vi "3d_aircraft.vi"(4 "RH Aileron":dbl=-2.3415980339050293 format="%#.4f", 5 "Elevator":dbl(slide)=4.274326801300049 scale=-10.0..10.0, 6 "LH Aileron":dbl=1.756198525428772 format="%#.4f", 7 "Rudder":dbl(slide)=-0.13481126725673676 scale=-10.0..10.0, 8 "Heading (deg)":dbl(knob) scale=0.0..360.0, 9 "Roll (deg)":dbl(slide)=61.490421295166016 scale=-40.0..40.0, 10 "Pitch (deg)":dbl(slide)=-8.517632484436035 scale=-20.0..20.0, 11 "visual":refnum<k7>(container) caption="3D 파라미터형 표면") -> ()   [LabVIEW 2015]
uses:
  <vilib>/express/express arith-compare/Formula/XNode/ExpressFormulaBlockNode.xnode
  <vilib>/Platform/NI_3dgraph.lvlib
panel:
  in  "Rudder z":dbl[][](array[numeric])=[[0.0, 0.0, 0.0, 0.0], [0.0, 0.4, 0.4, 0.0], [0.0, 1.1, 1.1, 0.0], [0.0, 1.5, 1.5, 0.0], [0.0, 1.4, 1.4, 0.0], [0.0, -1.4, -1.4, 0.0], [0.0, -1.5, -1.5, 0.0], [0.0, -1.1, -1.1, 0.0], [0.0, -0.4, -0.4, 0.0], [0.0, 0.0, 0.0, 0.0]]
  in  "Rudder y":dbl[][](array[numeric])=[[0.8, 7.0, 14.0, 21.0], [0.6, 7.0, 14.0, 21.0], [0.4, 7.0, 14.0, 21.0], [0.2, 7.0, 14.0, 21.0], [0.0, 7.0, 14.0, 21.0], [0.0, 7.0, 14.0, 21.0], [0.2, 7.0, 14.0, 21.0], [0.4, 7.0, 14.0, 21.0], [0.6, 7.0, 14.0, 21.0], [0.8, 7.0, 14.0, 21.0]]
  in  "Rudder x":dbl[][](array[numeric])=[[5.0, 5.0, 5.0, 5.0], [4.6667, 4.6667, 4.6667, 4.6667], [2.5, 2.5, 2.5, 2.5], [0.8333, 0.8333, 0.8333, 0.8333], [0.0, 0.0, 0.0, 0.0], [0.0, 0.0, 0.0, 0.0], [0.8333, 0.8333, 0.8333, 0.8333], [2.5, 2.5, 2.5, 2.5], [4.6667, 4.6667, 4.6667, 4.6667], [5.0, 5.0, 5.0, 5.0]]
  in  "Elevator z":dbl[][](array[numeric])=[[0.0, 0.0, 0.0, 0.0], [0.0, 0.4, 0.4, 0.0], [0.0, 1.1, 1.1, 0.0], [0.0, 1.5, 1.5, 0.0], [0.0, 1.4, 1.4, 0.0], [0.0, -1.4, -1.4, 0.0], [0.0, -1.5, -1.5, 0.0], [0.0, -1.1, -1.1, 0.0], [0.0, -0.4, -0.4, 0.0], [0.0, 0.0, 0.0, 0.0]]
  in  "Elevator y":dbl[][](array[numeric])=[[-12.0, -12.0, 12.0, 12.0], [-12.0, -12.0, 12.0, 12.0], [-12.0, -12.0, 12.0, 12.0], [-12.0, -12.0, 12.0, 12.0], [-12.0, -12.0, 12.0, 12.0], [-12.0, -12.0, 12.0, 12.0], [-12.0, -12.0, 12.0, 12.0], [-12.0, -12.0, 12.0, 12.0], [-12.0, -12.0, 12.0, 12.0], [-12.0, -12.0, 12.0, 12.0]]
  in  "Elevator x":dbl[][](array[numeric])=[[5.0, 5.0, 5.0, 5.0], [4.6667, 4.6667, 4.6667, 4.6667], [2.5, 2.5, 2.5, 2.5], [0.8333, 0.8333, 0.8333, 0.8333], [0.0, 0.0, 0.0, 0.0], [0.0, 0.0, 0.0, 0.0], [0.8333, 0.8333, 0.8333, 0.8333], [2.5, 2.5, 2.5, 2.5], [4.6667, 4.6667, 4.6667, 4.6667], [5.0, 5.0, 5.0, 5.0]]
  in  "Aileron z":dbl[][](array[numeric])=[[0.0, 0.0, 0.0, 0.0], [0.0, 0.3276, 0.3276, 0.0], [0.0, 0.5994, 0.5994, 0.0], [0.0, 1.0388, 1.0388, 0.0], [0.0, 1.3762, 1.3762, 0.0], [0.0, -0.2418, -0.2418, 0.0], [0.0, -0.1612, -0.1612, 0.0], [0.0, -0.0806, -0.0806, 0.0], [0.0, -0.0402, -0.0402, 0.0], [0.0, 0.0, 0.0, 0.0]]
  in  "Aileron y":dbl[][](array[numeric])=[[0.0, 0.0, 56.0, 56.0], [0.0, 0.0, 56.0, 56.0], [0.0, 0.0, 56.0, 56.0], [0.0, 0.0, 56.0, 56.0], [0.0, 0.0, 56.0, 56.0], [0.0, 0.0, 56.0, 56.0], [0.0, 0.0, 56.0, 56.0], [0.0, 0.0, 56.0, 56.0], [0.0, 0.0, 56.0, 56.0], [0.0, 0.0, 56.0, 56.0]]
  in  "Aileron x":dbl[][](array[numeric])=[[6.0, 6.0, 6.0, 6.0], [5.0, 5.0, 5.0, 5.0], [4.0, 4.0, 4.0, 4.0], [2.0, 2.0, 2.0, 2.0], [0.09999999999999964, 0.09999999999999964, 0.09999999999999964, 0.09999999999999964], [0.09999999999999964, 0.09999999999999964, 0.09999999999999964, 0.09999999999999964], [2.0, 2.0, 2.0, 2.0], [4.0, 4.0, 4.0, 4.0], [5.0, 5.0, 5.0, 5.0], [6.0, 6.0, 6.0, 6.0]]
  in  "Body z":dbl[][](array[numeric])=[[0.0, 0.0, 0.0, 0.0, 0.0, 0.0, 0.0, 0.0, 0.0], [-0.5, 1.0, 1.0, 20.0, 22.0, 20.0, 1.0, 1.0, -0.5], [-0.5, 1.5, 1.5, 20.0, 22.0, 20.0, 1.5, 1.5, -0.5], [-0.5, 1.0, 1.0, 8.0, 10.0, 8.0, 1.0, 1.0, -0.5], [-1.5, 0.0, 0.0, 3.0, 5.0, 3.0, 0.0, 0.0, -1.5], [-2.0, 0.0, 0.0, 0.0, 0.0, 0.0, 0.0, 0.0, -2.0], [-3.0, -0.276, -0.276, -0.276, -0.276, -0.276, -0.276, -0.276, -2.638], [-4.0, -0.4618, -0.4618, -0.4618, -0.4618, -0.4618, -0.4618, -0.4618, -3.2309], [-5.0, -0.5474, -0.5474, -0.5474, -0.5474, -0.5474, -0.5474, -0.5474, -3.5237], [-6.0, -0.5888, -0.5888, -0.5888, -0.5888, -0.5888, -0.5888, -0.5888, -3.7944], [-3.7418, -0.4836, -0.4836, -0.4836, -0.4836, -0.4836, -0.4836, -0.4836, -3.7418], [-3.6612, -0.3224, -0.3224, -0.3224, -0.3224, -0.3224, -0.3224, -0.3224, -3.6612], [-3.5806, -0.1612, -0.1612, -0.1612, -0.1612, -0.1612, -0.1612, -0.1612, -3.5806], [-3.5201, -0.0402, -0.0402, -0.0402, -0.0402, -0.0402, -0.0402, -0.0402, -3.5201], [-3.5, 0.0, 0.0, 0.0, 0.0, 0.0, 0.0, 0.0, -3.5], [-3.25, 0.0, 0.0, 0.0, 0.0, 0.0, 0.0, 0.0, -3.25], [-3.0, 0.0, 0.0, 0.0, 0.0, 0.0, 0.0, 0.0, -3.0], [-2.5, 0.0, 0.0, 0.0, 0.0, 0.0, 0.0, 0.0, -2.5], [-2.5, -5.0, -5.0, -5.0, -5.0, -5.0, -5.0, -5.0, -2.5], [-3.0, -6.0, -6.0, -6.0, -6.0, -6.0, -6.0, -6.0, -3.0], [-3.25, -6.5, -6.5, -6.5, -6.5, -6.5, -6.5, -6.5, -3.25], [-3.5, -7.0, -7.0, -7.0, -7.0, -7.0, -7.0, -7.0, -3.5], [-3.5201, -7.0, -7.0, -7.0, -7.0, -7.0, -7.0, -7.0, -3.5201], [-3.5806, -7.0, -7.0, -7.0, -7.0, -7.0, -7.0, -7.0, -3.5806], [-3.6612, -7.0, -7.0, -7.0, -7.0, -7.0, -7.0, -7.0, -3.6612], [-3.7418, -7.0, -7.0, -7.0, -7.0, -7.0, -7.0, -7.0, -3.7418], [-2.5, -7.0, -7.0, -7.0, -7.0, -7.0, -7.0, -7.0, -2.5], [-2.5, -7.0, -7.0, -7.0, -7.0, -7.0, -7.0, -7.0, -2.5], [-2.0, -7.0, -7.0, -7.0, -7.0, -7.0, -7.0, -7.0, -2.0], [-0.5, -7.0, -7.0, -7.0, -7.0, -7.0, -7.0, -7.0, -0.5], [-0.5, -6.5, -6.5, -6.5, -6.5, -6.5, -6.5, -6.5, -0.5], [-0.5, -3.5, -3.5, -3.5, -3.5, -3.5, -3.5, -3.5, -0.5], [-0.5, -2.0, -2.0, -2.0, -2.0, -2.0, -2.0, -2.0, -0.5], [-0.5, -2.5, -2.5, -2.5, -2.5, -2.5, -2.5, -2.5, -0.5], [-0.5, -2.0, -2.0, -2.0, -2.0, -2.0, -2.0, -2.0, -0.5], [0.0, 0.0, 0.0, 0.0, 0.0, 0.0, 0.0, 0.0, 0.0]]
  in  "Body y":dbl[][](array[numeric])=[[-12.0, -12.0, -2.0, -1.0, 0.0, 1.0, 2.0, 12.0, 12.0], [-12.0, -12.0, -2.0, -1.0, 0.0, 1.0, 2.0, 12.0, 12.0], [-12.0, -12.0, -2.0, -1.5, 0.0, 1.5, 2.0, 12.0, 12.0], [-2.0, -2.0, -2.5, -1.5, 0.0, 1.5, 2.5, 2.0, 2.0], [-2.5, -2.5, -3.0, -1.5, 0.0, 1.5, 3.0, 2.5, 2.5], [-2.799999999999997, -2.799999999999997, -3.0, -1.5, 0.0, 1.5, 3.0, 2.799999999999997, 2.799999999999997], [-3.0, -3.0, -3.0, -1.0, 0.0, 1.0, 3.0, 3.0, 3.0], [-3.0, -3.0, -3.0, -1.0, 0.0, 1.0, 3.0, 3.0, 3.0], [-3.0, -3.0, -3.0, -1.0, 0.0, 1.0, 3.0, 3.0, 3.0], [-3.0, -3.0, -3.0, -1.0, 0.0, 1.0, 3.0, 3.0, 3.0], [-3.0, -3.0, -3.0, -1.0, 0.0, 1.0, 3.0, 3.0, 3.0], [-3.0, -3.0, -3.0, -1.0, 0.0, 1.0, 3.0, 3.0, 3.0], [-3.0, -3.0, -3.0, -1.0, 0.0, 1.0, 3.0, 3.0, 3.0], [-3.0, -3.0, -3.0, -1.0, 0.0, 1.0, 3.0, 3.0, 3.0], [-3.0, -3.0, -3.0, -1.0, 0.0, 1.0, 3.0, 3.0, 3.0], [-3.0, -3.0, -3.0, -1.0, 0.0, 1.0, 3.0, 3.0, 3.0], [-2.5, -2.5, -2.5, -1.0, 0.0, 1.0, 2.5, 2.5, 2.5], [-2.0, -2.0, -2.0, -1.0, 0.0, 1.0, 2.0, 2.0, 2.0], [-2.0, -2.0, -2.0, -1.0, 0.0, 1.0, 2.0, 2.0, 2.0], [-2.5, -2.5, -2.5, -1.0, 0.0, 1.0, 2.5, 2.5, 2.5], [-3.0, -3.0, -3.0, -1.0, 0.0, 1.0, 3.0, 3.0, 3.0], [-3.0, -3.0, -3.0, -1.0, 0.0, 1.0, 3.0, 3.0, 3.0], [-3.0, -3.0, -3.0, -1.0, 0.0, 1.0, 3.0, 3.0, 3.0], [-3.0, -3.0, -3.0, -1.0, 0.0, 1.0, 3.0, 3.0, 3.0], [-3.0, -3.0, -3.0, -1.0, 0.0, 1.0, 3.0, 3.0, 3.0], [-3.0, -3.0, -3.0, -1.0, 0.0, 1.0, 3.0, 3.0, 3.0], [-3.0, -3.0, -3.0, -1.0, 0.0, 1.0, 3.0, 3.0, 3.0], [-3.0, -3.0, -3.0, -1.0, 0.0, 1.0, 3.0, 3.0, 3.0], [-3.0, -3.0, -3.0, -1.0, 0.0, 1.0, 3.0, 3.0, 3.0], [-3.0, -3.0, -3.0, -1.0, 0.0, 1.0, 3.0, 3.0, 3.0], [-2.799999999999997, -2.799999999999997, -3.0, -1.0, 0.0, 1.0, 3.0, 2.799999999999997, 2.799999999999997], [-2.5, -2.5, -3.0, -1.0, 0.0, 1.0, 3.0, 2.5, 2.5], [-2.0, -2.0, -2.5, -1.0, 0.0, 1.0, 2.5, 2.0, 2.0], [-12.0, -12.0, -3.0, -1.0, 0.0, 1.0, 3.0, 12.0, 12.0], [-12.0, -12.0, -3.0, -1.0, 0.0, 1.0, 3.0, 12.0, 12.0], [-12.0, -12.0, -3.0, -1.0, 0.0, 1.0, 3.0, 12.0, 12.0]]
  in  "Body x":dbl[][](array[numeric])=[[45.0, 45.0, 45.0, 45.0, 45.0, 45.0, 45.0, 45.0, 45.0], [45.0, 45.0, 45.0, 45.0, 45.0, 45.0, 45.0, 45.0, 45.0], [41.5, 42.5, 42.5, 42.5, 42.5, 42.5, 42.5, 42.5, 41.5], [34.0, 35.0, 35.0, 35.0, 35.0, 35.0, 35.0, 35.0, 34.0], [24.0, 25.0, 25.0, 25.0, 25.0, 25.0, 25.0, 25.0, 24.0], [14.0, 15.0, 15.0, 15.0, 15.0, 15.0, 15.0, 15.0, 14.0], [6.0, 7.0, 7.0, 7.0, 7.0, 7.0, 7.0, 7.0, 6.0], [4.0, 5.0, 5.0, 5.0, 5.0, 5.0, 5.0, 5.0, 4.0], [3.0, 3.0, 3.0, 3.0, 3.0, 3.0, 3.0, 3.0, 3.0], [1.0, 1.0, 1.0, 1.0, 1.0, 1.0, 1.0, 1.0, 1.0], [-1.0, -1.0, -1.0, -1.0, -1.0, -1.0, -1.0, -1.0, -1.0], [-2.0, -2.0, -2.0, -2.0, -2.0, -2.0, -2.0, -2.0, -2.0], [-3.0, -3.0, -3.0, -3.0, -3.0, -3.0, -3.0, -3.0, -3.0], [-3.5, -3.5, -3.5, -3.5, -3.5, -3.5, -3.5, -3.5, -3.5], [-6.0, -6.0, -6.0, -6.0, -6.0, -6.0, -6.0, -6.0, -6.0], [-10.0, -10.0, -10.0, -10.0, -10.0, -10.0, -10.0, -10.0, -10.0], [-15.0, -15.0, -15.0, -15.0, -15.0, -15.0, -15.0, -15.0, -15.0], [-20.0, -20.0, -20.0, -20.0, -20.0, -20.0, -20.0, -20.0, -20.0], [-20.0, -20.0, -20.0, -20.0, -20.0, -20.0, -20.0, -20.0, -20.0], [-15.0, -15.0, -15.0, -15.0, -15.0, -15.0, -15.0, -15.0, -15.0], [-10.0, -10.0, -10.0, -10.0, -10.0, -10.0, -10.0, -10.0, -10.0], [-6.0, -6.0, -6.0, -6.0, -6.0, -6.0, -6.0, -6.0, -6.0], [-3.5, -3.5, -3.5, -3.5, -3.5, -3.5, -3.5, -3.5, -3.5], [-3.0, -3.0, -3.0, -3.0, -3.0, -3.0, -3.0, -3.0, -3.0], [-2.0, -2.0, -2.0, -2.0, -2.0, -2.0, -2.0, -2.0, -2.0], [-1.0, -1.0, -1.0, -1.0, -1.0, -1.0, -1.0, -1.0, -1.0], [1.0, 1.0, 1.0, 1.0, 1.0, 1.0, 1.0, 1.0, 1.0], [3.0, 3.0, 3.0, 3.0, 3.0, 3.0, 3.0, 3.0, 3.0], [4.0, 5.0, 5.0, 5.0, 5.0, 5.0, 5.0, 5.0, 4.0], [6.0, 7.0, 7.0, 7.0, 7.0, 7.0, 7.0, 7.0, 6.0], [14.0, 15.0, 15.0, 15.0, 15.0, 15.0, 15.0, 15.0, 14.0], [24.0, 25.0, 25.0, 25.0, 25.0, 25.0, 25.0, 25.0, 24.0], [34.0, 35.0, 35.0, 35.0, 35.0, 35.0, 35.0, 35.0, 34.0], [41.5, 42.5, 42.5, 42.5, 42.5, 42.5, 42.5, 42.5, 41.5], [45.0, 45.0, 45.0, 45.0, 45.0, 45.0, 45.0, 45.0, 45.0], [45.0, 45.0, 45.0, 45.0, 45.0, 45.0, 45.0, 45.0, 45.0]]
  in  "Wing z":dbl[][](array[numeric])=[[0.0, 0.0, 0.0, 0.0, 0.0, 0.0, 0.0, 0.0], [0.0, 0.3276, 0.3276, 0.3276, 0.3276, 0.3276, 0.3276, 0.0], [0.0, 0.5994, 0.5994, 0.5994, 0.5994, 0.5994, 0.5994, 0.0], [0.0, 1.0388, 1.0388, 1.0388, 1.0388, 1.0388, 1.0388, 0.0], [0.0, 1.3762, 1.3762, 1.3762, 1.3762, 1.3762, 1.3762, 0.0], [0.0, 1.6196, 1.6196, 1.6196, 1.6196, 1.6196, 1.6196, 0.0], [0.0, 1.773, 1.773, 1.773, 1.773, 1.773, 1.773, 0.0], [0.0, 1.8284, 1.8284, 1.8284, 1.8284, 1.8284, 1.8284, 0.0], [0.0, 1.7718, 1.7718, 1.7718, 1.7718, 1.7718, 1.7718, 0.0], [0.0, 1.5912, 1.5912, 1.5912, 1.5912, 1.5912, 1.5912, 0.0], [0.0, 1.431, 1.431, 1.431, 1.431, 1.431, 1.431, 0.0], [0.0, 1.2026, 1.2026, 1.2026, 1.2026, 1.2026, 1.2026, 0.0], [0.0, 1.0444, 1.0444, 1.0444, 1.0444, 1.0444, 1.0444, 0.0], [0.0, 0.8482, 0.8482, 0.8482, 0.8482, 0.8482, 0.8482, 0.0], [0.0, 0.5782, 0.5782, 0.5782, 0.5782, 0.5782, 0.5782, 0.0], [0.0, 0.39, 0.39, 0.39, 0.39, 0.39, 0.39, 0.0], [0.0, 0.0, 0.0, 0.0, 0.0, 0.0, 0.0, 0.0], [0.0, 0.0, 0.0, 0.0, 0.0, 0.0, 0.0, 0.0], [0.0, -0.276, -0.276, -0.276, -0.276, -0.276, -0.276, 0.0], [0.0, -0.3658, -0.3658, -0.3658, -0.3658, -0.3658, -0.3658, 0.0], [0.0, -0.4618, -0.4618, -0.4618, -0.4618, -0.4618, -0.4618, 0.0], [0.0, -0.5116, -0.5116, -0.5116, -0.5116, -0.5116, -0.5116, 0.0], [0.0, -0.5474, -0.5474, -0.5474, -0.5474, -0.5474, -0.5474, 0.0], [0.0, -0.579, -0.579, -0.579, -0.579, -0.579, -0.579, 0.0], [0.0, -0.5888, -0.5888, -0.5888, -0.5888, -0.5888, -0.5888, 0.0], [0.0, -0.5562, -0.5562, -0.5562, -0.5562, -0.5562, -0.5562, 0.0], [0.0, -0.4836, -0.4836, -0.4836, -0.4836, -0.4836, -0.4836, 0.0], [0.0, -0.403, -0.403, -0.403, -0.403, -0.403, -0.403, 0.0], [0.0, -0.3224, -0.3224, -0.3224, -0.3224, -0.3224, -0.3224, 0.0], [0.0, -0.2418, -0.2418, -0.2418, -0.2418, -0.2418, -0.2418, 0.0], [0.0, -0.2418, -0.2418, -0.1612, -0.1612, -0.2418, -0.2418, 0.0], [0.0, -0.2418, -0.2418, -0.0806, -0.0806, -0.2418, -0.2418, 0.0], [0.0, -0.2418, -0.2418, -0.0402, -0.0402, -0.2418, -0.2418, 0.0], [0.0, -0.2418, -0.2418, 0.0, 0.0, -0.2418, -0.2418, 0.0]]
  in  "Wing y":dbl[][](array[numeric])=[[-60.0, -60.0, -4.0, -3.0, 3.0, 4.0, 60.0, 60.0], [-60.0, -60.0, -4.0, -3.0, 3.0, 4.0, 60.0, 60.0], [-60.0, -60.0, -4.0, -3.0, 3.0, 4.0, 60.0, 60.0], [-60.0, -60.0, -4.0, -3.0, 3.0, 4.0, 60.0, 60.0], [-60.0, -60.0, -4.0, -3.0, 3.0, 4.0, 60.0, 60.0], [-60.0, -60.0, -4.0, -3.0, 3.0, 4.0, 60.0, 60.0], [-60.0, -60.0, -4.0, -3.0, 3.0, 4.0, 60.0, 60.0], [-60.0, -60.0, -4.0, -3.0, 3.0, 4.0, 60.0, 60.0], [-60.0, -60.0, -4.0, -3.0, 3.0, 4.0, 60.0, 60.0], [-60.0, -60.0, -4.0, -3.0, 3.0, 4.0, 60.0, 60.0], [-60.0, -60.0, -4.0, -3.0, 3.0, 4.0, 60.0, 60.0], [-60.0, -60.0, -4.0, -3.0, 3.0, 4.0, 60.0, 60.0], [-60.0, -60.0, -4.0, -3.0, 3.0, 4.0, 60.0, 60.0], [-60.0, -60.0, -4.0, -3.0, 3.0, 4.0, 60.0, 60.0], [-60.0, -60.0, -4.0, -3.0, 3.0, 4.0, 60.0, 60.0], [-60.0, -60.0, -4.0, -3.0, 3.0, 4.0, 60.0, 60.0], [-60.0, -60.0, -4.0, -3.0, 3.0, 4.0, 60.0, 60.0], [-60.0, -60.0, -4.0, -3.0, 3.0, 4.0, 60.0, 60.0], [-60.0, -60.0, -4.0, -3.0, 3.0, 4.0, 60.0, 60.0], [-60.0, -60.0, -4.0, -3.0, 3.0, 4.0, 60.0, 60.0], [-60.0, -60.0, -4.0, -3.0, 3.0, 4.0, 60.0, 60.0], [-60.0, -60.0, -4.0, -3.0, 3.0, 4.0, 60.0, 60.0], [-60.0, -60.0, -4.0, -3.0, 3.0, 4.0, 60.0, 60.0], [-60.0, -60.0, -4.0, -3.0, 3.0, 4.0, 60.0, 60.0], [-60.0, -60.0, -4.0, -3.0, 3.0, 4.0, 60.0, 60.0], [-60.0, -60.0, -4.0, -3.0, 3.0, 4.0, 60.0, 60.0], [-60.0, -60.0, -4.0, -3.0, 3.0, 4.0, 60.0, 60.0], [-60.0, -60.0, -4.0, -3.0, 3.0, 4.0, 60.0, 60.0], [-60.0, -60.0, -4.0, -3.0, 3.0, 4.0, 60.0, 60.0], [-60.0, -60.0, -4.0, -3.0, 3.0, 4.0, 60.0, 60.0], [-60.0, -60.0, -4.0, -3.0, 3.0, 4.0, 60.0, 60.0], [-60.0, -60.0, -4.0, -3.0, 3.0, 4.0, 60.0, 60.0], [-60.0, -60.0, -4.0, -3.0, 3.0, 4.0, 60.0, 60.0]]
  in  "Wing x":dbl[][](array[numeric])=[[8.9, 8.9, 8.9, 15.0, 15.0, 8.9, 8.9, 8.9], [8.9, 8.9, 8.9, 13.5, 13.5, 8.9, 8.9, 8.9], [8.9, 8.9, 8.9, 12.0, 12.0, 8.9, 8.9, 8.9], [8.9, 8.9, 8.9, 10.5, 10.5, 8.9, 8.9, 8.9], [8.9, 8.9, 8.9, 9.0, 9.0, 8.9, 8.9, 8.9], [7.0, 7.0, 7.0, 7.0, 7.0, 7.0, 7.0, 7.0], [5.0, 5.0, 5.0, 5.0, 5.0, 5.0, 5.0, 5.0], [3.0, 3.0, 3.0, 3.0, 3.0, 3.0, 3.0, 3.0], [1.0, 1.0, 1.0, 1.0, 1.0, 1.0, 1.0, 1.0], [-1.0, -1.0, -1.0, -1.0, -1.0, -1.0, -1.0, -1.0], [-2.0, -2.0, -2.0, -2.0, -2.0, -2.0, -2.0, -2.0], [-3.0, -3.0, -3.0, -3.0, -3.0, -3.0, -3.0, -3.0], [-3.5, -3.5, -3.5, -3.5, -3.5, -3.5, -3.5, -3.5], [-4.0, -4.0, -4.0, -4.0, -4.0, -4.0, -4.0, -4.0], [-4.5, -4.5, -4.5, -4.5, -4.5, -4.5, -4.5, -4.5], [-4.75, -4.75, -4.75, -4.75, -4.75, -4.75, -4.75, -4.75], [-5.0, -5.0, -5.0, -5.0, -5.0, -5.0, -5.0, -5.0], [-5.0, -5.0, -5.0, -5.0, -5.0, -5.0, -5.0, -5.0], [-4.75, -4.75, -4.75, -4.75, -4.75, -4.75, -4.75, -4.75], [-4.5, -4.5, -4.5, -4.5, -4.5, -4.5, -4.5, -4.5], [-4.0, -4.0, -4.0, -4.0, -4.0, -4.0, -4.0, -4.0], [-3.5, -3.5, -3.5, -3.5, -3.5, -3.5, -3.5, -3.5], [-3.0, -3.0, -3.0, -3.0, -3.0, -3.0, -3.0, -3.0], [-2.0, -2.0, -2.0, -2.0, -2.0, -2.0, -2.0, -2.0], [-1.0, -1.0, -1.0, -1.0, -1.0, -1.0, -1.0, -1.0], [1.0, 1.0, 1.0, 1.0, 1.0, 1.0, 1.0, 1.0], [3.0, 3.0, 3.0, 3.0, 3.0, 3.0, 3.0, 3.0], [5.0, 5.0, 5.0, 5.0, 5.0, 5.0, 5.0, 5.0], [7.0, 7.0, 7.0, 7.0, 7.0, 7.0, 7.0, 7.0], [8.9, 8.9, 8.9, 9.0, 9.0, 8.9, 8.9, 8.9], [8.9, 8.9, 8.9, 10.5, 10.5, 8.9, 8.9, 8.9], [8.9, 8.9, 8.9, 12.0, 12.0, 8.9, 8.9, 8.9], [8.9, 8.9, 8.9, 13.5, 13.5, 8.9, 8.9, 8.9], [8.9, 8.9, 8.9, 15.0, 15.0, 8.9, 8.9, 8.9]]
  out "i":i32
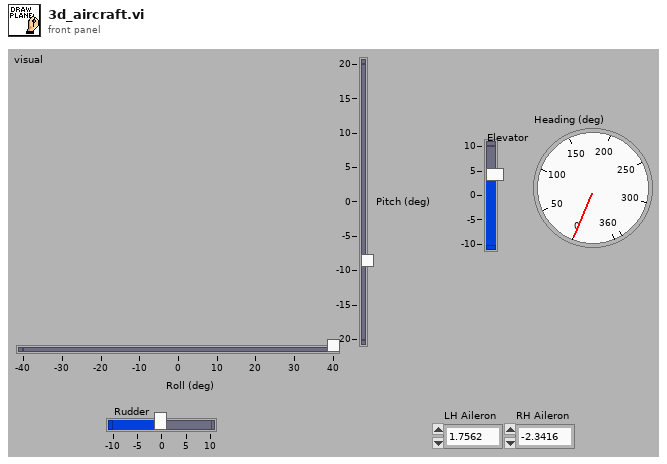
[diagram p1: front panel]
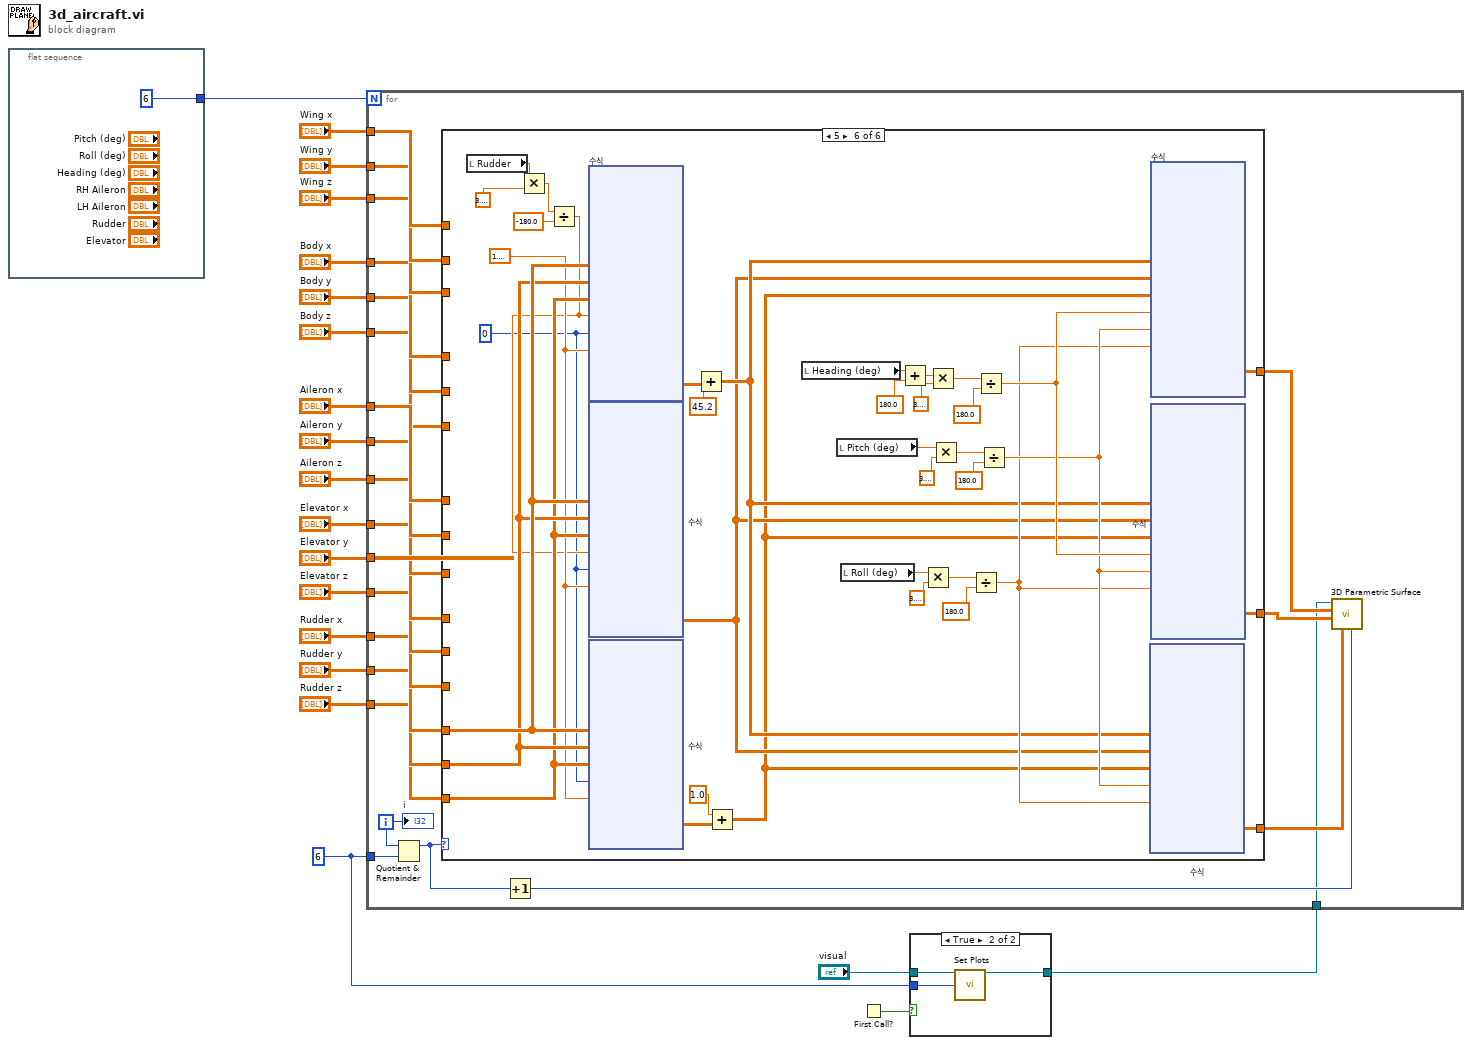
[diagram p0: block diagram]
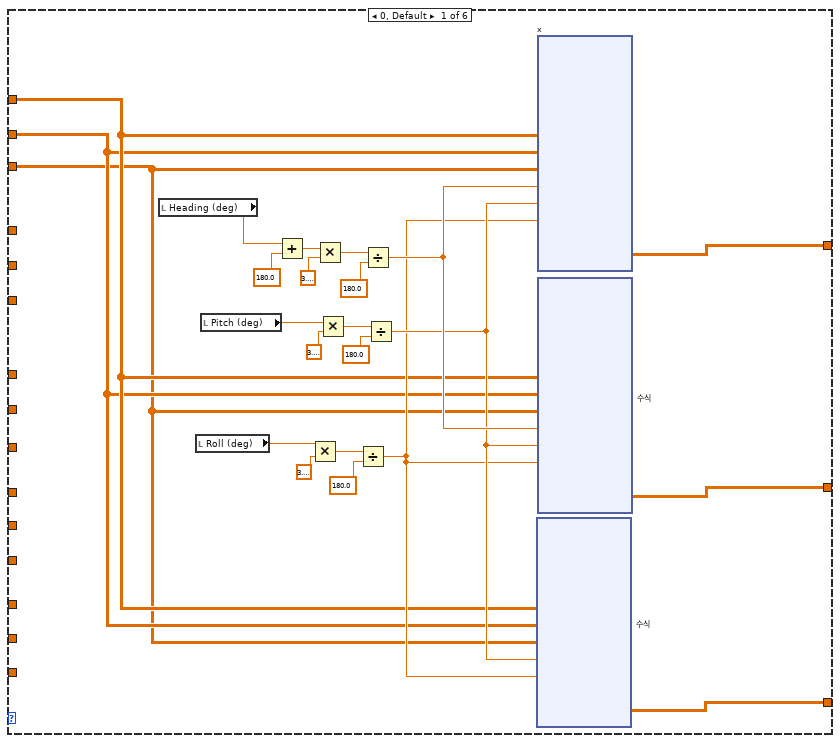
[diagram p3: hidden frame]
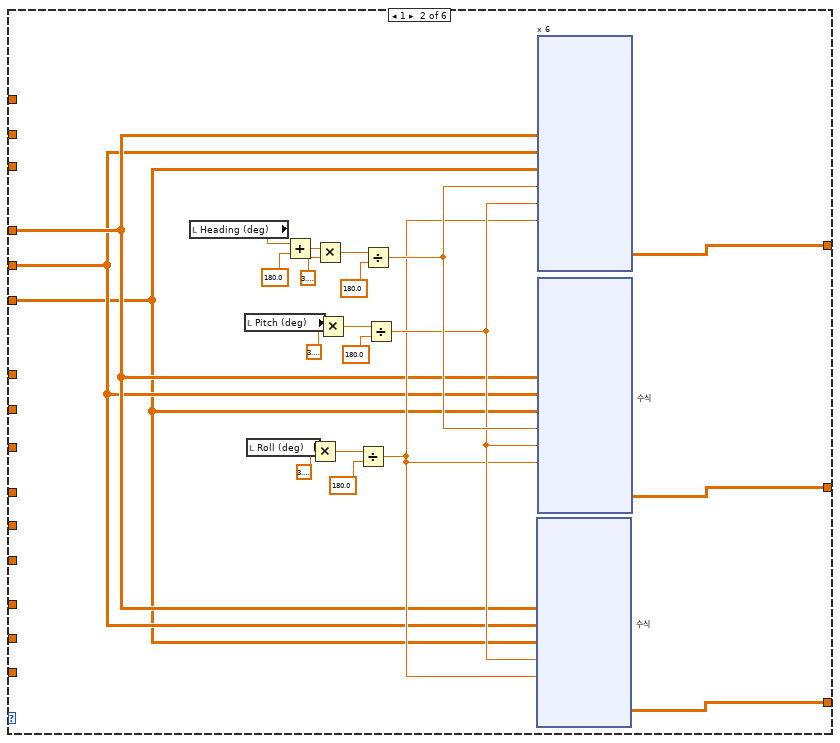
[diagram p4: hidden frame]
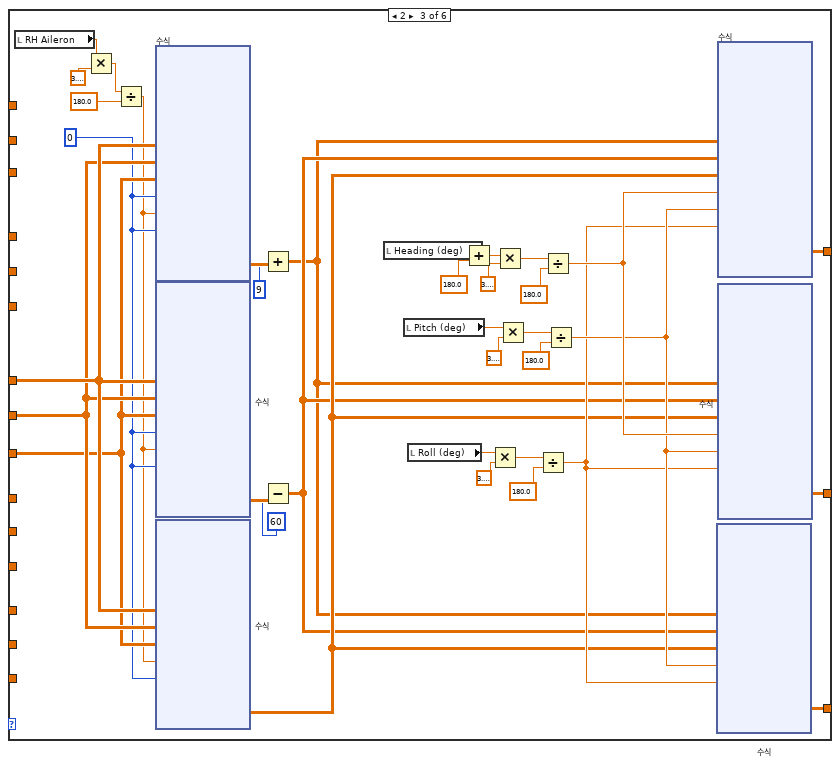
[diagram p5: hidden frame]
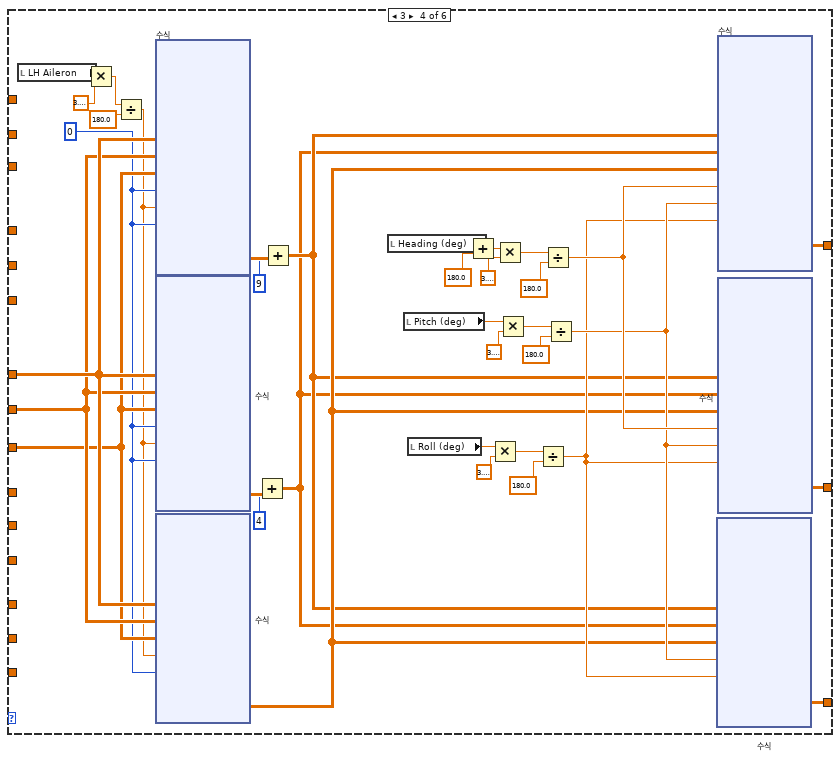
[diagram p6: hidden frame]
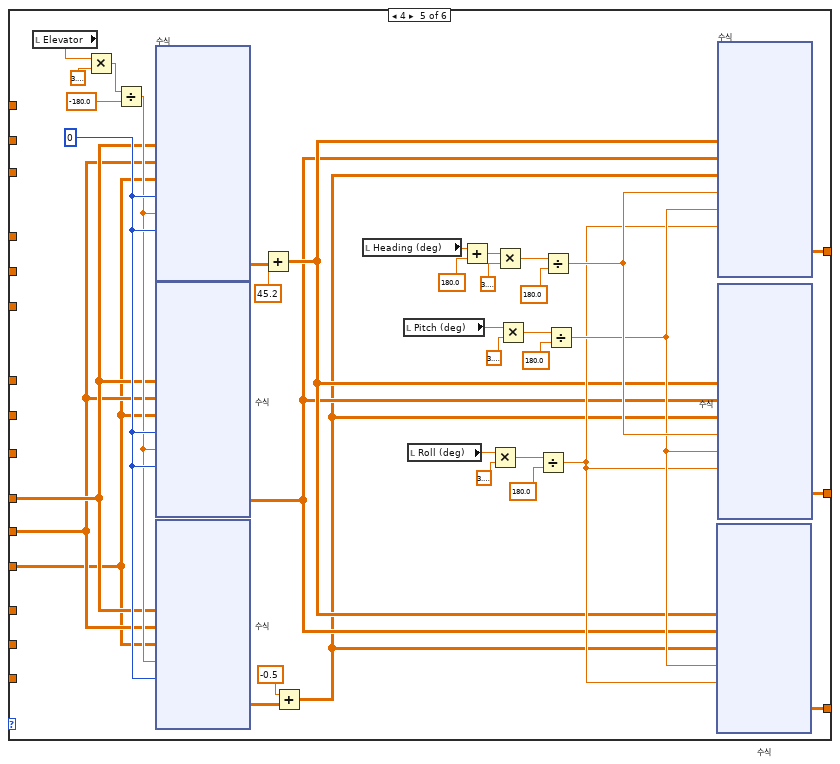
[diagram p7: hidden frame]
diagram:
  w19 = 6 ("y")
  n1 = flat-sequence {
    tunnel: [6] -> w2
    frame #0 {
    }
  }
  n2 = First Call?() -> (First Call?: T/F=w1:bool)
  n3 = case shown="True" w1 {
    tunnel: "visual" -> [w22 w25]
    tunnel: w19 -> [_ w24]
    tunnel: [w22 w23] -> w18
    frame False {
    }
    frame True {
      n4 = call <vilib>:"Set Plots.vi"("3D graph"=w25, "# of plots(1)"=w24) -> ("3D graph out"=w23:refnum<k7>)  [unwired: 1 in, 12 out]
    }
  }
  n5 = for {
    N: w2 -> [_]
    tunnel: "Wing x" -> [w48]
    tunnel: "Wing y" -> [w47]
    tunnel: "Wing z" -> [w46]
    tunnel: "Aileron x" -> [w45]
    tunnel: "Aileron y" -> [w44]
    tunnel: "Aileron z" -> [w43]
    tunnel: w19 -> [w36]
    tunnel: w18 -> [w35]
    tunnel: "Body x" -> [w34]
    tunnel: "Body y" -> [w33]
    tunnel: "Body z" -> [w32]
    tunnel: "Elevator x" -> [w31]
    tunnel: "Elevator y" -> [w30]
    tunnel: "Elevator z" -> [w29]
    tunnel: "Rudder x" -> [w28]
    tunnel: "Rudder y" -> [w27]
    tunnel: "Rudder z" -> [w26]
    i -> [w42]
    n6 = Quotient & Remainder(x=w42, y=w36) -> (x-y*floor(x/y)=w38:i32)  [unwired: 1 out]
    n7 = case shown="5" w38 {
      tunnel: [w71 w198 w338 w582 w826 w1071] -> w39
      tunnel: [w70 w197 w337 w581 w825 w1070] -> w41
      tunnel: [w69 w196 w336 w580 w824 w1069] -> w40
      tunnel: w48 -> [w56 _ _ _ _ _]
      tunnel: w47 -> [w55 _ _ _ _ _]
      tunnel: w46 -> [w54 _ _ _ _ _]
      tunnel: w45 -> [_ _ w323 w567 _ _]
      tunnel: w44 -> [_ _ w322 w566 _ _]
      tunnel: w43 -> [_ _ w321 w565 _ _]
      tunnel: w34 -> [_ w183 _ _ _ _]
      tunnel: w33 -> [_ w182 _ _ _ _]
      tunnel: w32 -> [_ w181 _ _ _ _]
      tunnel: w31 -> [_ _ _ _ w803 _]
      tunnel: w30 -> [_ _ _ _ w802 _]
      tunnel: w29 -> [_ _ _ _ w801 _]
      tunnel: w28 -> [_ _ _ _ _ w1047]
      tunnel: w27 -> [_ _ _ _ _ w1046]
      tunnel: w26 -> [_ _ _ _ _ w1045]
      frame 0, Default {
        n8 = local read "Heading (deg)"() -> (w51:dbl)
        n9 = local read "Roll (deg)"() -> (w50:dbl)
        n10 = local read "Pitch (deg)"() -> (w49:dbl)
        n11 = Add(x=w51, y=180.0) -> (x+y=w52:dbl)
        n12 = Multiply(x=w50, y=3.141592653589793) -> (x*y=w62:dbl)
        n13 = Multiply(x=w52, y=3.141592653589793) -> (x*y=w68:dbl)
        n14 = Multiply(x=w49, y=3.141592653589793) -> (x*y=w65:dbl)
        n15 = Divide(x=w62, y=180.0) -> (x/y=w57:dbl)
        n16 = Divide(x=w68, y=180.0) -> (x/y=w59:dbl)
        n17 = Divide(x=w65, y=180.0) -> (x/y=w58:dbl)
        n18 = xnode "수식"("x0"=w56, "y0"=w55, "z0"=w54, "pitch"=w58, "roll"=w57) -> ("결과"=w69:dbl[][])  [unwired: 2 in, 1 out]
        n19 = xnode("x0"=w56, "y0"=w55, "z0"=w54, "yaw"=w59, "pitch"=w58, "roll"=w57) -> ("결과"=w71:dbl[][])  [unwired: 2 in, 1 out]
        n20 = xnode "수식"("x0"=w56, "y0"=w55, "z0"=w54, "yaw"=w59, "pitch"=w58, "roll"=w57) -> ("결과"=w70:dbl[][])  [unwired: 2 in, 1 out]
      }
      frame 1 {
        n21 = local read "Heading (deg)"() -> (w178:dbl)
        n22 = local read "Pitch (deg)"() -> (w176:dbl)
        n23 = local read "Roll (deg)"() -> (w177:dbl)
        n24 = Add(x=w178, y=180.0) -> (x+y=w179:dbl)
        n25 = Multiply(x=w177, y=3.141592653589793) -> (x*y=w189:dbl)
        n26 = Multiply(x=w179, y=3.141592653589793) -> (x*y=w195:dbl)
        n27 = Multiply(x=w176, y=3.141592653589793) -> (x*y=w192:dbl)
        n28 = Divide(x=w189, y=180.0) -> (x/y=w184:dbl)
        n29 = Divide(x=w195, y=180.0) -> (x/y=w186:dbl)
        n30 = Divide(x=w192, y=180.0) -> (x/y=w185:dbl)
        n31 = xnode "수식"("x0"=w183, "y0"=w182, "z0"=w181, "pitch"=w185, "roll"=w184) -> ("결과"=w196:dbl[][])  [unwired: 2 in, 1 out]
        n32 = xnode ("x 6")("x0"=w183, "y0"=w182, "z0"=w181, "yaw"=w186, "pitch"=w185, "roll"=w184) -> ("결과"=w198:dbl[][])  [unwired: 2 in, 1 out]
        n33 = xnode "수식"("x0"=w183, "y0"=w182, "z0"=w181, "yaw"=w186, "pitch"=w185, "roll"=w184) -> ("결과"=w197:dbl[][])  [unwired: 2 in, 1 out]
      }
      frame 2 {
        w320 = 0
        n34 = local read "RH Aileron"() -> (w305:dbl)
        n35 = Multiply(x=w305, y=3.141592653589793) -> (x*y=w312:dbl)
        n36 = Divide(x=w312, y=180.0) -> (x/y=w309:dbl)
        n37 = xnode "수식"("x0"=w323, "y0"=w322, "z0"=w321, "yaw"=w320, "pitch"=w309, "roll"=w320) -> ("결과"=w315:dbl[][])  [unwired: 2 in, 1 out]
        n38 = xnode "수식"("x0"=w323, "y0"=w322, "z0"=w321, "yaw"=w320, "pitch"=w309, "roll"=w320) -> ("결과"=w318:dbl[][])  [unwired: 2 in, 1 out]
        n39 = xnode "수식"("x0"=w323, "y0"=w322, "z0"=w321, "pitch"=w309, "roll"=w320) -> ("결과"=w319:dbl[][])  [unwired: 2 in, 1 out]
        n40 = Add(x=w315, y=9) -> (x+y=w314:dbl[][])
        n41 = Subtract(x=w318, y=60) -> (x-y=w317:dbl[][])
        n42 = local read "Heading (deg)"() -> (w306:dbl)
        n43 = local read "Pitch (deg)"() -> (w303:dbl)
        n44 = local read "Roll (deg)"() -> (w304:dbl)
        n45 = Add(x=w306, y=180.0) -> (x+y=w307:dbl)
        n46 = Multiply(x=w304, y=3.141592653589793) -> (x*y=w329:dbl)
        n47 = Multiply(x=w307, y=3.141592653589793) -> (x*y=w335:dbl)
        n48 = Multiply(x=w303, y=3.141592653589793) -> (x*y=w332:dbl)
        n49 = Divide(x=w329, y=180.0) -> (x/y=w324:dbl)
        n50 = Divide(x=w335, y=180.0) -> (x/y=w326:dbl)
        n51 = Divide(x=w332, y=180.0) -> (x/y=w325:dbl)
        n52 = xnode "수식"("x0"=w314, "y0"=w317, "z0"=w319, "pitch"=w325, "roll"=w324) -> ("결과"=w336:dbl[][])  [unwired: 2 in, 1 out]
        n53 = xnode "수식"("x0"=w314, "y0"=w317, "z0"=w319, "yaw"=w326, "pitch"=w325, "roll"=w324) -> ("결과"=w338:dbl[][])  [unwired: 2 in, 1 out]
        n54 = xnode "수식"("x0"=w314, "y0"=w317, "z0"=w319, "yaw"=w326, "pitch"=w325, "roll"=w324) -> ("결과"=w337:dbl[][])  [unwired: 2 in, 1 out]
      }
      frame 3 {
        w564 = 0
        n55 = local read "LH Aileron"() -> (w549:dbl)
        n56 = Multiply(x=w549, y=3.141592653589793) -> (x*y=w559:dbl)
        n57 = Divide(x=w559, y=180.0) -> (x/y=w556:dbl)
        n58 = xnode "수식"("x0"=w567, "y0"=w566, "z0"=w565, "yaw"=w564, "pitch"=w556, "roll"=w564) -> ("결과"=w562:dbl[][])  [unwired: 2 in, 1 out]
        n59 = xnode "수식"("x0"=w567, "y0"=w566, "z0"=w565, "yaw"=w564, "pitch"=w556, "roll"=w564) -> ("결과"=w555:dbl[][])  [unwired: 2 in, 1 out]
        n60 = xnode "수식"("x0"=w567, "y0"=w566, "z0"=w565, "pitch"=w556, "roll"=w564) -> ("결과"=w563:dbl[][])  [unwired: 2 in, 1 out]
        n61 = Add(x=w555, y=4) -> (x+y=w554:dbl[][])
        n62 = Add(x=w562, y=9) -> (x+y=w561:dbl[][])
        n63 = local read "Heading (deg)"() -> (w550:dbl)
        n64 = local read "Pitch (deg)"() -> (w547:dbl)
        n65 = local read "Roll (deg)"() -> (w548:dbl)
        n66 = Add(x=w550, y=180.0) -> (x+y=w551:dbl)
        n67 = Multiply(x=w548, y=3.141592653589793) -> (x*y=w573:dbl)
        n68 = Multiply(x=w551, y=3.141592653589793) -> (x*y=w579:dbl)
        n69 = Multiply(x=w547, y=3.141592653589793) -> (x*y=w576:dbl)
        n70 = Divide(x=w573, y=180.0) -> (x/y=w568:dbl)
        n71 = Divide(x=w579, y=180.0) -> (x/y=w570:dbl)
        n72 = Divide(x=w576, y=180.0) -> (x/y=w569:dbl)
        n73 = xnode "수식"("x0"=w561, "y0"=w554, "z0"=w563, "pitch"=w569, "roll"=w568) -> ("결과"=w580:dbl[][])  [unwired: 2 in, 1 out]
        n74 = xnode "수식"("x0"=w561, "y0"=w554, "z0"=w563, "yaw"=w570, "pitch"=w569, "roll"=w568) -> ("결과"=w582:dbl[][])  [unwired: 2 in, 1 out]
        n75 = xnode "수식"("x0"=w561, "y0"=w554, "z0"=w563, "yaw"=w570, "pitch"=w569, "roll"=w568) -> ("결과"=w581:dbl[][])  [unwired: 2 in, 1 out]
      }
      frame 4 {
        w811 = 0
        n76 = local read "Elevator"() -> (w793:dbl)
        n77 = Multiply(x=w793, y=3.141592653589793) -> (x*y=w807:dbl)
        n78 = Divide(x=w807, y=-180.0) -> (x/y=w804:dbl)
        n79 = xnode "수식"("x0"=w803, "y0"=w802, "z0"=w801, "yaw"=w811, "pitch"=w804, "roll"=w811) -> ("결과"=w810:dbl[][])  [unwired: 2 in, 1 out]
        n80 = xnode "수식"("x0"=w803, "y0"=w802, "z0"=w801, "yaw"=w811, "pitch"=w804, "roll"=w811) -> ("결과"=w800:dbl[][])  [unwired: 2 in, 1 out]
        n81 = xnode "수식"("x0"=w803, "y0"=w802, "z0"=w801, "pitch"=w804, "roll"=w811) -> ("결과"=w799:dbl[][])  [unwired: 2 in, 1 out]
        n82 = Add(x=w810, y=45.2 ("숫자형")) -> (x+y=w809:dbl[][])
        n83 = Add(x=-0.5 ("숫자형"), y=w799) -> (x+y=w798:dbl[][])
        n84 = local read "Heading (deg)"() -> (w795:dbl)
        n85 = local read "Pitch (deg)"() -> (w792:dbl)
        n86 = local read "Roll (deg)"() -> (w791:dbl)
        n87 = Add(x=w795, y=180.0) -> (x+y=w794:dbl)
        n88 = Multiply(x=w791, y=3.141592653589793) -> (x*y=w817:dbl)
        n89 = Multiply(x=w794, y=3.141592653589793) -> (x*y=w823:dbl)
        n90 = Multiply(x=w792, y=3.141592653589793) -> (x*y=w820:dbl)
        n91 = Divide(x=w817, y=180.0) -> (x/y=w812:dbl)
        n92 = Divide(x=w823, y=180.0) -> (x/y=w814:dbl)
        n93 = Divide(x=w820, y=180.0) -> (x/y=w813:dbl)
        n94 = xnode "수식"("x0"=w809, "y0"=w800, "z0"=w798, "pitch"=w813, "roll"=w812) -> ("결과"=w824:dbl[][])  [unwired: 2 in, 1 out]
        n95 = xnode "수식"("x0"=w809, "y0"=w800, "z0"=w798, "yaw"=w814, "pitch"=w813, "roll"=w812) -> ("결과"=w826:dbl[][])  [unwired: 2 in, 1 out]
        n96 = xnode "수식"("x0"=w809, "y0"=w800, "z0"=w798, "yaw"=w814, "pitch"=w813, "roll"=w812) -> ("결과"=w825:dbl[][])  [unwired: 2 in, 1 out]
      }
      frame 5 {
        w1043 = 1.5707963267948966
        w1041 = 0
        n97 = local read "Rudder"() -> (w1037:dbl)
        n98 = Multiply(x=w1037, y=3.141592653589793) -> (x*y=w1053:dbl)
        n99 = Divide(x=w1053, y=-180.0) -> (x/y=w1042:dbl)
        n100 = xnode "수식"("x0"=w1047, "y0"=w1046, "z0"=w1045, "yaw"=w1042, "pitch"=w1041, "roll"=w1043) -> ("결과"=w1056:dbl[][])  [unwired: 2 in, 1 out]
        n101 = xnode "수식"("x0"=w1047, "y0"=w1046, "z0"=w1045, "yaw"=w1042, "pitch"=w1041, "roll"=w1043) -> ("결과"=w1051:dbl[][])  [unwired: 2 in, 1 out]
        n102 = xnode "수식"("x0"=w1047, "y0"=w1046, "z0"=w1045, "pitch"=w1041, "roll"=w1043) -> ("결과"=w1050:dbl[][])  [unwired: 2 in, 1 out]
        n103 = Add(x=w1056, y=45.2 ("숫자형")) -> (x+y=w1055:dbl[][])
        n104 = Add(x=1.0 ("숫자형 2"), y=w1050) -> (x+y=w1049:dbl[][])
        n105 = local read "Heading (deg)"() -> (w1039:dbl)
        n106 = local read "Pitch (deg)"() -> (w1036:dbl)
        n107 = local read "Roll (deg)"() -> (w1035:dbl)
        n108 = Add(x=w1039, y=180.0) -> (x+y=w1038:dbl)
        n109 = Multiply(x=w1035, y=3.141592653589793) -> (x*y=w1062:dbl)
        n110 = Multiply(x=w1038, y=3.141592653589793) -> (x*y=w1068:dbl)
        n111 = Multiply(x=w1036, y=3.141592653589793) -> (x*y=w1065:dbl)
        n112 = Divide(x=w1062, y=180.0) -> (x/y=w1057:dbl)
        n113 = Divide(x=w1068, y=180.0) -> (x/y=w1059:dbl)
        n114 = Divide(x=w1065, y=180.0) -> (x/y=w1058:dbl)
        n115 = xnode "수식"("x0"=w1055, "y0"=w1051, "z0"=w1049, "pitch"=w1058, "roll"=w1057) -> ("결과"=w1069:dbl[][])  [unwired: 2 in, 1 out]
        n116 = xnode "수식"("x0"=w1055, "y0"=w1051, "z0"=w1049, "yaw"=w1059, "pitch"=w1058, "roll"=w1057) -> ("결과"=w1071:dbl[][])  [unwired: 2 in, 1 out]
        n117 = xnode "수식"("x0"=w1055, "y0"=w1051, "z0"=w1049, "yaw"=w1059, "pitch"=w1058, "roll"=w1057) -> ("결과"=w1070:dbl[][])  [unwired: 2 in, 1 out]
      }
    }
    n118 = Increment(x=w38) -> (x+1=w37:i32)
    n119 = call <vilib>:"3D Parametric Surface.vi"("plot number (1)"=w37, "z matrix"=w40, "y matrix"=w41, "x matrix"=w39, "3D graph"=w35) -> ()  [unwired: 5 in, 2 out]
    "i" <- w42
  }
